vi "PH_Revolver-GUI_6P.Evt Call Select Position.vi"(0 "i ref in":refnum<vi>, 1 "Revolver Instance":string, 3 "Wanted Position":T1 items=["unknown", "Position 0", "Position 60", "Position 120", "Position 180", "Position 240", "Position 300", "moving"], 5 "error in":errorcluster) -> (14 "i ref out":refnum<vi>, 19 "error out":errorcluster)   [LabVIEW 2014, in "PH_Revolver-GUI_6P.lvlib"]
uses:
  PH_Revolver-GUI_6P.lvlib
  PH_Revolver-GUI_6P.Position.ctl
  CSCore/CSSystem/CoreLib/CoreLib.short 2 byte array.vi
  CSCore/CSSystem/CoreLib/CoreLib.lvlib
  CSCore/BaseProcess/BaseProcess.lvlib
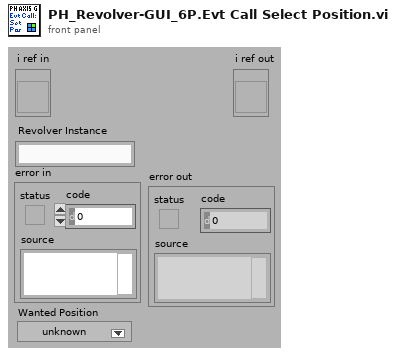
[diagram p1: front panel]
types:
  T1 = typedef "PH_Revolver-GUI_6P.lvlib/PH_Revolver-GUI_6P.Position.ctl" = u16
  T2 = typedef "CoreDefs.rawDataType.ctl" = i8[]
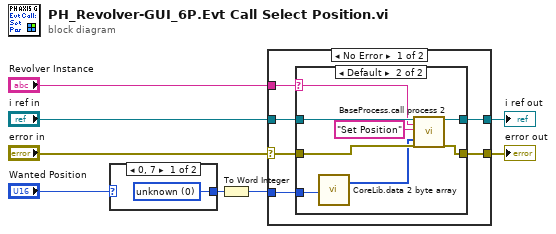
[diagram p0: block diagram]
diagram:
  n1 = case shown="0, 7" "Wanted Position" {
    selector: "Wanted Position" -> [_ w10]
    tunnel: [w9 w10] -> w1
    frame 0, 7 {
      w9 = T1 0 items=["unknown", "Position 0", "Position 60", "Position 120", "Position 180", "Position 240", "Position 300", "moving"] ("Wanted Position")
    }
    frame Default {
    }
  }
  n2 = To Word Integer(number=w1) -> (16bit integer=w3:i16)
  n3 = case shown="No Error" "error in" {
    selector: "error in" -> [w12 w27]
    tunnel: [w16 w27] -> w5
    tunnel: "Revolver Instance" -> [w11 _]
    tunnel: "i ref in" -> [w15 w28]
    tunnel: [w14 w28] -> w7
    tunnel: w3 -> [w13 _]
    frame No Error {
      n4 = case shown="Default" w11 {
        selector: w11 -> [_ w19]
        tunnel: [w18 w26] -> w16
        tunnel: w12 -> [w18 w24]
        tunnel: w15 -> [w17 w23]
        tunnel: [w17 w22] -> w14
        tunnel: w13 -> [_ w21]
        frame "N/A" {
        }
        frame Default {
          n5 = call-poly "CoreLib.data 2 byte array.vi"("i16"=w21) -> ("byteArray out"=w20:T2)  [unwired: 18 in]
          n6 = call "BaseProcess.call process 2.vi"("i ref in"=w23, "Object"=w19, "Selector"="Set Position", "Data"=w20, "error in (no error)"=w24) -> ("i ref out"=w22:refnum<vi>, "error out"=w26:errorcluster)  [unwired: 13 in]
        }
      }
    }
    frame Error {
    }
  }
  "i ref out" <- w7
  "error out" <- w5
